vi "Read Warning Log Data.vi"(8 "error in":errorcluster, 11 "Fault Handler in":refnum<class "Fault Handler.lvclass">) -> (0 "error out":errorcluster, 3 "Fault Handler out":refnum<class "Fault Handler.lvclass">)   [LabVIEW 2023, in "Fault Handler.lvlib" / "Fault Handler.lvclass"]
uses:
  Library/Fault Handler.lvclass
  Library/Fault Handler.lvclass/Fault Handler.ctl
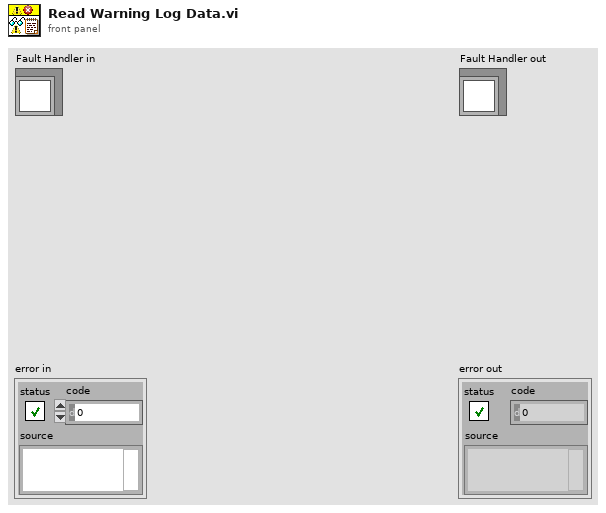
[diagram p1: front panel]
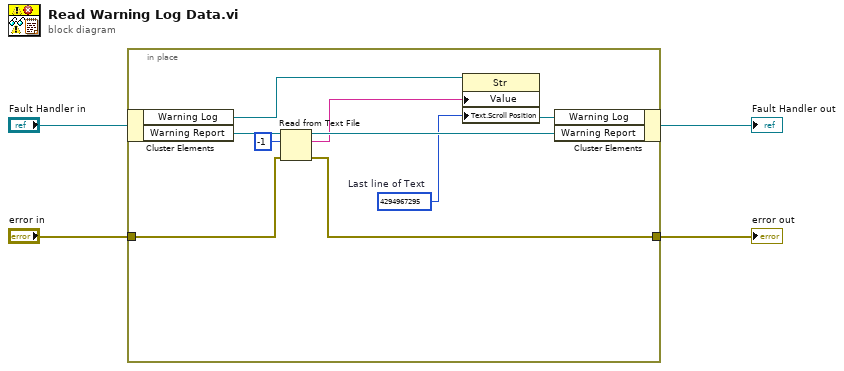
[diagram p0: block diagram]
diagram:
  n1 = in-place {
    in-place-border: "error in" -> [w10]
    in-place-border: [w9] -> w1
    w5 = u32 4294967295  # Last line of Text
    n2 = in-place-cluster #1("Fault Handler in") -> ("Warning Log"=w8:refnum<vi>, "Warning Report"=w13:refnum<file>)
    n3 = Read from Text File(file (use dialog)=w13, count=-1, error in=w10) -> (refnum out=w12:refnum<file>, text=w6:string, error out=w9:errorcluster)  [unwired: 1 in, 1 out]
    n4 = property class="Str"(reference=w8, "Value"=w6, "Text.Scroll Position"=w5) -> (reference out=w7:refnum<vi>)  [unwired: 1 in, 1 out]
    n5 = in-place-cluster #1("Warning Log"=w7, "Warning Report"=w12) -> (→"Fault Handler out":refnum<class "Fault Handler.lvclass">)
  }
  "error out" <- w1
